vi "GUI_TektronixDPOSimple_multidev.vi"() -> ()   [LabVIEW 2013]
uses:
  Shared/GUI_Template/GUI_master/tcp_new_data_event.ctl
  Shared/GUI_Template/GUI_master/tcp new data cluster.ctl
panel:
  out "Device name new event":string
  in  "This Application":refnum<vi>
  in  "Refresh Button":bool
  in  "Select device":string(combo)="StagingPXIFast1"
  in  "Cluster":T1 caption="BELLA_TEK_DSO"
  in  "stop":bool
  out "GUIdevice 1":string="BELLA_TEK_DSO"
  out "error IO 2":errorcluster
  in  "insert tag":bool=TRUE
  out "tcp data event":T2
  in  "UDP error message":string
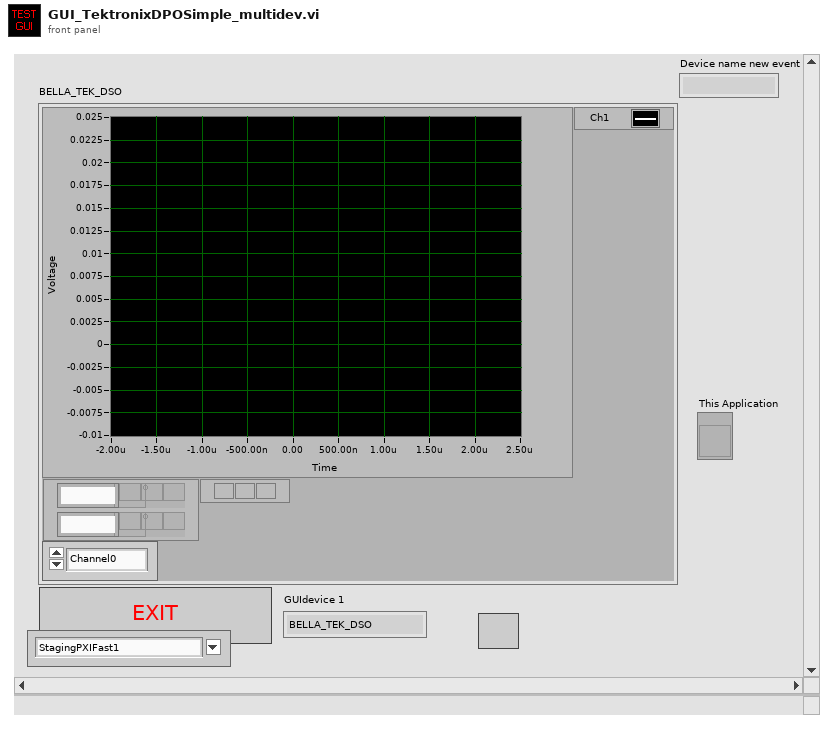
[diagram p1: front panel]
types:
  T1 = cluster{"scopeTraceGUI::1":waveform(dbl)[], "Channel::1":enum16{"Channel0", "Channel1", "Channel2", "Channel3"}}
  T2 = typedef "tcp_new_data_event.ctl" = refnum<user-event>
  T3 = typedef "tcp new data cluster.ctl" = cluster{"EventEnum":enum16{"new data", "connection status update"}, "Device name":string}
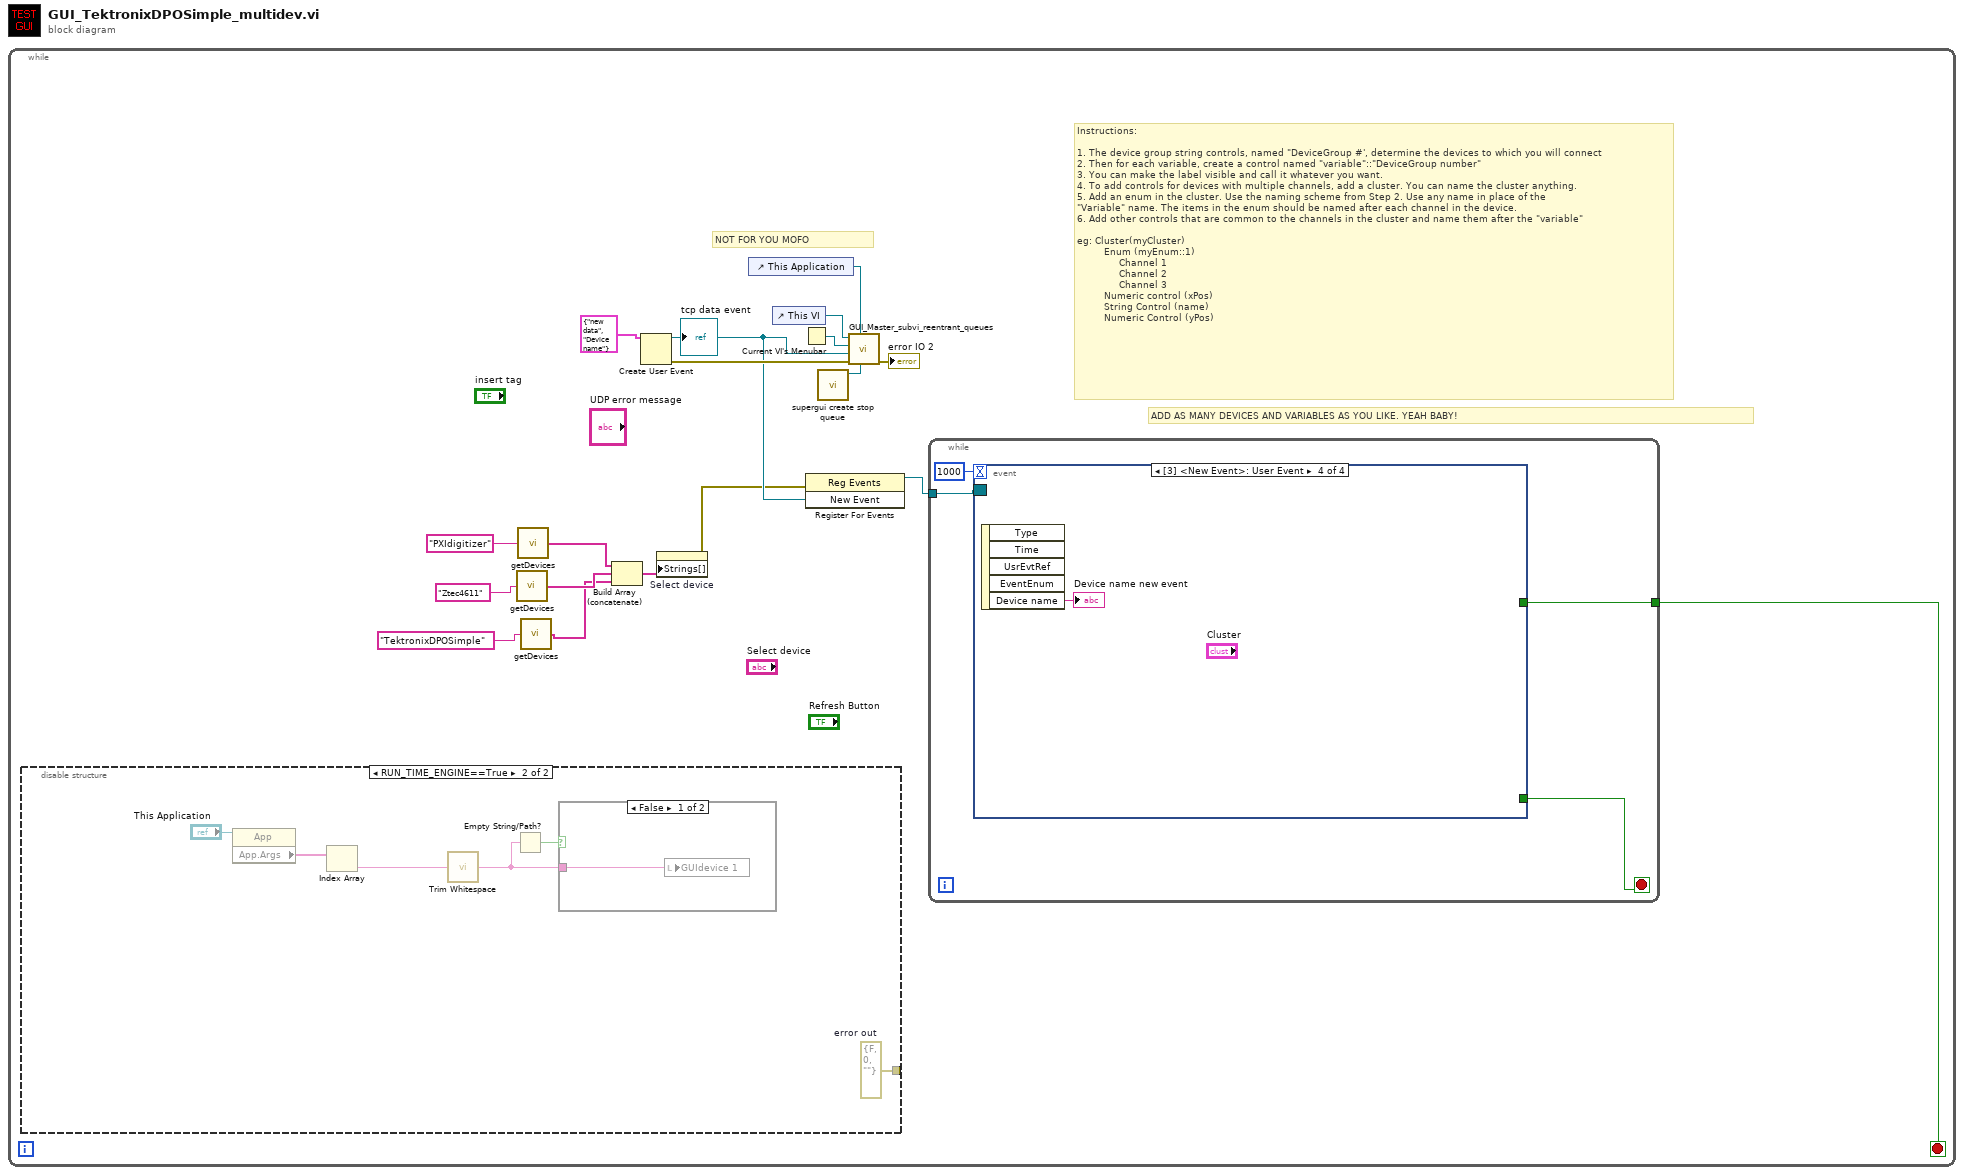
[diagram p0: block diagram]
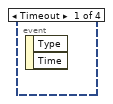
[diagram p4: hidden frame]
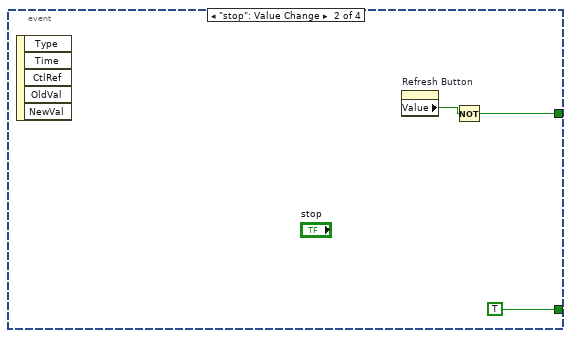
[diagram p5: hidden frame]
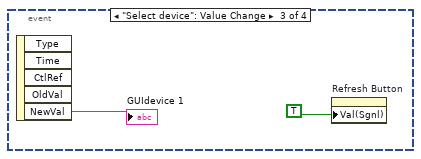
[diagram p6: hidden frame]
diagram:
  n1 = while {
    stop <- w2 stop-if-true
    # "Instructions:\n\n1. The device group string controls, named \"DeviceGroup #', determine the devices to which you will connect\n2. Then for each variable, create a control named \"variable\"::\"DeviceGroup number\"\n3. You can make the label visible and call it whatever you want.\n4. To add controls for devices with multiple channels, add a cluster. You can name the cluster anything.\n5. Add an enum in the cluster. Use the naming scheme from Step 2. Use any name in place of the \n\"Variable\" name. The items in the enum should be named after each channel in the device. \n6. Add other controls that are common to the channels in the cluster and name them after the \"variable\"\n\neg: Cluster(myCluster)\n         Enum (myEnum::1)\n              Channel 1 \n              Channel 2\n              Channel 3\n         Numeric control (xPos)\n         String Control (name)\n         Numeric Control (yPos)"
    # "ADD AS MANY DEVICES AND VARIABLES AS YOU LIKE. YEAH BABY!"
    # "NOT FOR YOU MOFO"
    n2 = disable-structure shown="RUN_TIME_ENGINE==True" {
      disable-tunnel: [_ w19] -> _
      frame condition #0 (active) {
      }
      frame condition #1 {
        w19 = errorcluster {"status"=FALSE, "code"=0, "source"=""}  # error out
        n3 = property class="App"(reference="This Application") -> ("App.Args"=w24:string[])  [unwired: 1 in, 2 out]
        n4 = Index Array(array=w24) -> (element=w21:string)  [unwired: 1 in]
        n5 = call <vilib>:"Trim Whitespace.vi"("string"=w21) -> ("trimmed string"=w20:string)  [unwired: 1 in]
        n6 = Empty String/Path?(string/path=w20) -> (empty?=w22:bool)
        n7 = case shown="False" w22 {
          tunnel: w20 -> [w25 _]
          frame False {
            n8 = local write "GUIdevice 1"(w25) -> ()
          }
          frame True {
          }
        }
      }
    }
    n9 = call "getDevices.vi"("Device Class"="Ztec4611") -> ("All Devices"=w7:string[])
    n10 = call "getDevices.vi"("Device Class"="PXIdigitizer") -> ("All Devices"=w8:string[])
    n11 = call "getDevices.vi"("Device Class"="TektronixDPOSimple") -> ("All Devices"=w3:string[])
    n12 = Build Array (concatenate)(w8, w7, w3) -> (w6:string[])
    n13 = Create User Event(user event datatype=T3 {"EventEnum"=enum."new data", "Device name"="Device name"} ("New Event")) -> (user event=w12:refnum<user-event>, error out=w18:errorcluster)  [unwired: 1 in]
    "tcp data event" <- w12
    n14 = property on="Select device" class="CmbBox"("Strings[]"=w6) -> (error out=w5:errorcluster)  [unwired: 2 in, 1 out]
    n15 = control-ref of="This Application"() -> (w13:refnum<vi>)
    n16 = control-ref of="This VI"() -> (w15:refnum<vi>)
    n17 = Current VI's Menubar() -> (w16:refnum<k9>)
    n18 = register-events(error in=w5, w12) -> (reference out=w11:refnum<event-registration>)  [unwired: 1 in, 1 out]
    n19 = call "supergui create stop queue.vi"() -> ("STOP Queue out"=w1:refnum<queue>)  [unwired: 11 in]
    n20 = call "GUI_Master_subvi_reentrant_queues.vi"("STOP Queue in"=w1, "This Application"=w13, "error in (no error)"=w18, "tcp data event"=w12, "Caller menu reference"=w16, "Caller VI ref"=w15) -> ("error out"=→"error IO 2":errorcluster)  [unwired: 5 in]
    n21 = while {
      tunnel: w11 -> [w29]
      tunnel: [w26] -> w2
      stop <- w27 stop-if-true
      n22 = event shown="[3] <New Event>: User Event" {
        selector: w29 -> [_ _ _ _]
        dyn-events: _ -> [_ _ _ _]
        timeout: 1000 -> [_ _ _ _]
        tunnel: [_ TRUE _ _] -> w27
        tunnel: [_ w30 _ _] -> w26
        event Timeout {
          n23 = event-data() -> ()  [unwired: 1 in, 2 out]
        }
        event "stop": Value Change {
          n24 = event-data() -> ()  [unwired: 1 in, 5 out]
          n25 = property on="Refresh Button" class="Bool (strict)"() -> ("Value"=w31:bool)  [unwired: 2 in, 2 out]
          n26 = Not(x=w31) -> (.not. x?=w30:bool)
        }
        event "Select device": Value Change {
          n27 = event-data() -> ("NewVal"=→"GUIdevice 1":string)  [unwired: 1 in, 4 out]
          n28 = property on="Refresh Button" class="Bool (strict)"("Val(Sgnl)"=TRUE ("Value (Signaling)")) -> ()  [unwired: 2 in, 2 out]
        }
        event User Event {
          n29 = event-data() -> ("Device name"=→"Device name new event":string)  [unwired: 1 in, 4 out]
        }
      }
    }
  }
